vi "Double FFT Mesurament (Max Bin detection - Control - Init Wave&Window - Snapshot - DoubleFFT) RT Test.vi"() -> ()   [LabVIEW 2014]
uses:
  <vilib>/Platform/TimedLoop/XDataNode/timing_clust.ctl
  <vilib>/Platform/TimedLoop/XDataNode/nitl_modes.ctl
  <vilib>/Platform/TimedLoop/XDataNode/wakeup.ctl
  <vilib>/FPGAPlugInAG/sbRIO-9636/niLvFpga_Open_sbRIO-9636.vi
  <vilib>/rvi/interface/common/dynamic/niFpgaDynamicAddResources.vi
  <vilib>/Utility/error.llb/Error Cluster From Error Code.vi
  <vilib>/rvi/errors/niLvFpgaAdjustHostInterfaceError.vi
  <vilib>/rvi/interface/common/niFpgaWaitOnOcc.vi
  <vilib>/FPGAPlugInAG/Dynamic/niLvFpga_Run_Dynamic.vi
  <vilib>/FPGAPlugInAG/Dynamic/niLvFpga_Abort_Dynamic.vi
  <vilib>/FPGAPlugInAG/Dynamic/niLvFpga_Reset_Dynamic.vi
  <vilib>/FPGAPlugInAG/Dynamic/niLvFpga_Close_Dynamic.vi
  <vilib>/rvi/interface/nirviOpenFPGA/nirviOpenFPGA.xnode
  FPGA Bitfiles/LaserDistanceSen_FPGATarget_DoubleFFTMesuram_TCh4DSruzm8.lvbitx
  FPGA Target/Test VIs/Double FFT Mesurament (Max Bin detection - Control - Init Wave&Window - Snapshot - DoubleFFT) test.vi
  <vilib>/rvi/interface/nirviReadWriteControl/nirviReadWriteControl.xnode
  <vilib>/rvi/interface/nirviMethod/nirviMethod.xnode
  <vilib>/Platform/TimedLoop/XDataNode/XDataNode.xnode
  <vilib>/rvi/interface/nirviCloseFPGA/nirviCloseFPGA.xnode
  <vilib>/FPGAPlugInAG/Dynamic/niLvFpga_ConfigureFifo_Dynamic.vi
  <vilib>/rvi/errors/niLvFpgaMergeErrorWithErrorCode.vi
  <vilib>/FPGAPlugInAG/Dynamic/niLvFpga_StartFifo_Dynamic.vi
  <vilib>/rvi/interface/Simulation/niFpgaSimulationCallBeginRW.vi
  <vilib>/FPGAPlugInAG/Dynamic/niLvFpga_ReadFifo_Dynamic.vi
  <vilib>/Platform/TimedLoop/XDataNode/XDNodeRunTimeDep.lvlib
  NiFpgaLv.dll
panel:
  out "Second FFT (bin)":dbl[](graph)
  out "Second Signal (points) - Rising Triangular":dbl[](graph)
  out "Elements Remaining FFT":u32
  out "Elements Remaining Signal":u32
  out "First FFT (bin)":dbl[](graph)
  out "First Signal (points) - Falling Triangular":dbl[](graph)
  in  "Snapshot":bool
  in  "Windowing":T1(ring)
  in  "first bin":i32=10
  in  "last bin":i32=255
  in  "lower limit 2":u32(slide)=677 scale=625.0..738.0
  in  "lower limit 1":u32(slide)=59 scale=0.0..113.0
  out "Detected Frequency Tone - (Hz)":dbl
  in  "stop":bool
  out "Max Bin":i32
  out "Max Amp":dbl format="%.2f"
  out "Prev Bin":i32
  out "Next Bin":i32
  out "Prev Amp":dbl format="%.2f"
  out "Next Amp":dbl format="%.2f"
  out "Interpolated Bin":dbl
  in  "Interpolation Method":T2(ring)=enum."Jain"
  # "WARNING:\nOnce pressed wait untill the end of operation"
  # "ONLINE parameter"
  # "OFFLINE parameters"
  # "Max Detection FFT bin range"
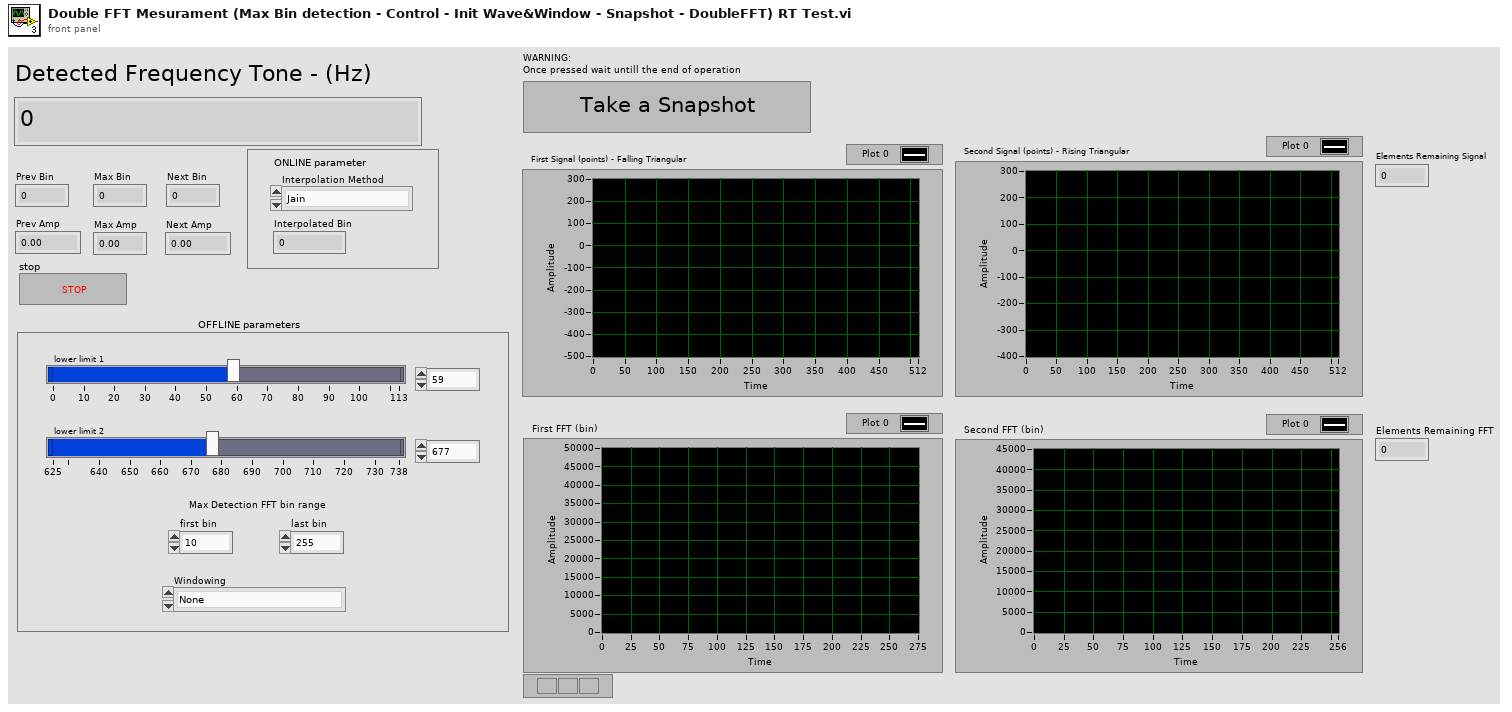
[diagram p1: front panel]
types:
  T1 = enum16{"None", "Hanning", "Hamming", "Blackman", "Blackman-Harris"}
  T2 = enum16{"Quadratic", "McLeodd", "Barycentric", "Jain"}
  T3 = typedef "XDNodeRunTimeDep.lvlib/timing_clust.ctl" = cluster{"Expected End [f-1]":u64, "Actual End [f-1]":u64, "Finished Late? [f-1]":bool, "Expected End [i-1]":u64, "Actual End [i-1]":u64, "Finished Late? [i-1]":bool, "Expected Start [i]":u64, "Actual Start [i]":u64, "Expected Start [f]":u64, "Actual Start [f]":u64, "Source Name":string, "Structure Name":string, "Period":i64, "Deadline":i64, "Offset":i64, "Start":i64, "Priority":i32, "Timeout":i32, "Mode":T4, "Wakeup Reason":T5, "Error":errorcluster, "Source Type":string, "Secondary Source Type":string, "Global End Time":u64, "Global Start Time":u64, "Frame Duration":u64, "Iteration Duration":u64, "Assigned CPU":i32, "I/O Scan Engine Mode":u32}
  T4 = typedef "XDNodeRunTimeDep.lvlib/nitl_modes.ctl" = enum32{"No Change", "Process missed periods, maintain original phase", "Discard missed periods, maintain original phase", "Process missed periods, ignore original phase", "Discard missed periods, ignore original phase"}
  T5 = typedef "XDNodeRunTimeDep.lvlib/wakeup.ctl" = enum32{"Normal", "Aborted", "Asynchronous wakeup", "Timing source error", "Timed loop error", "Timeout"}
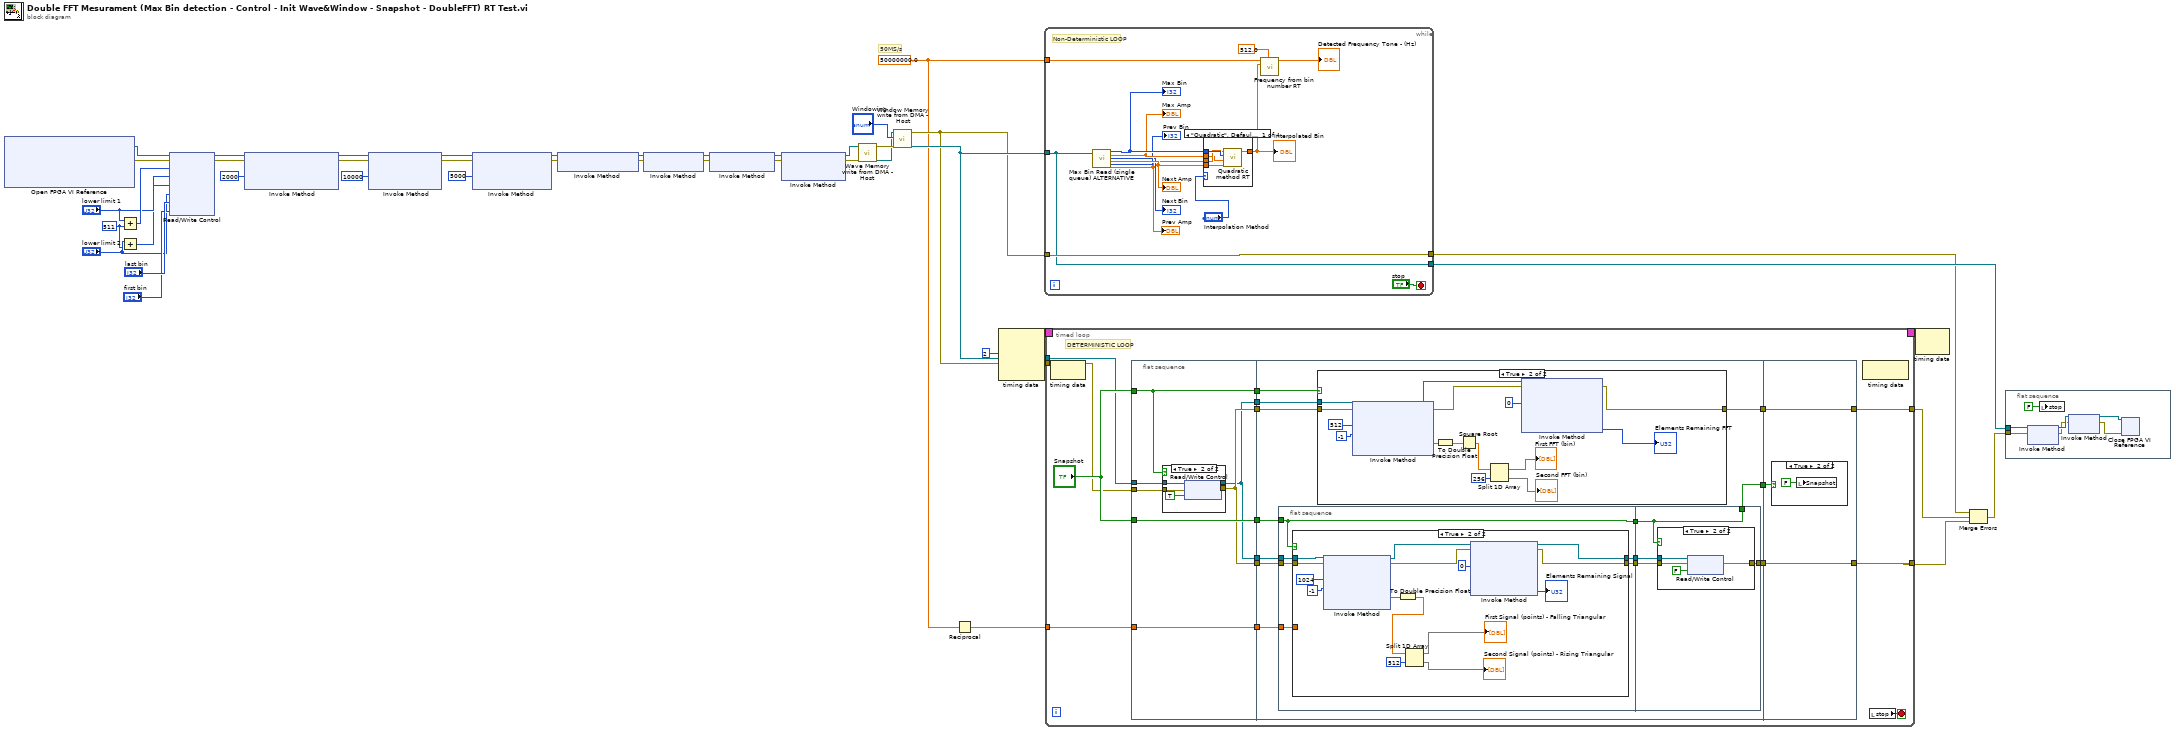
[diagram p0: block diagram]
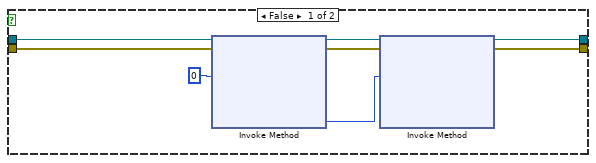
[diagram p3: hidden frame]
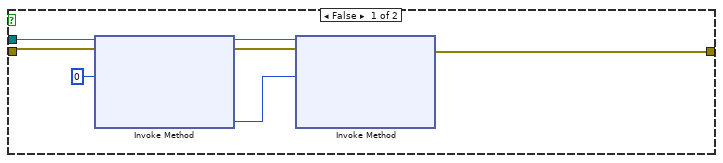
[diagram p5: hidden frame]
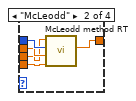
[diagram p7: hidden frame]
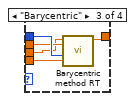
[diagram p8: hidden frame]
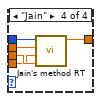
[diagram p9: hidden frame]
diagram:
  w37 = u32 511 ("y")
  w15 = 50000000.0 ("Sample Rate (S/s)")
  # "50MS/s"
  n1 = xnode "Open FPGA VI Reference"() -> ("FPGA VI Reference Out"=w36:refnum<k20>, "error out"=w35:errorcluster)  [unwired: 2 in]
  n2 = Add(x="lower limit 1", y=w37) -> (x+y=w41:u32)
  n3 = Add(x="lower limit 2", y=w37) -> (x+y=w39:u32)
  n4 = xnode "Read/Write Control"("FPGA VI Reference In"=w36, "error in"=w35, "upper limit 1"=w41, "upper limit 2"=w39, "lower limit 1"="lower limit 1", "lower limit 2"="lower limit 2", "last bin"="last bin", "first bin"="first bin") -> ("FPGA VI Reference Out"=w30:refnum<k20>, "error out"=w29:errorcluster)
  n5 = xnode "Invoke Method"("FPGA VI Reference In"=w30, "error in"=w29, "Requested Depth"=u32 2000) -> ("FPGA VI Reference Out"=w28:refnum<k20>, "error out"=w27:errorcluster)  [unwired: 1 out]
  n6 = xnode "Invoke Method"("FPGA VI Reference In"=w28, "error in"=w27, "Requested Depth"=u32 10000) -> ("FPGA VI Reference Out"=w26:refnum<k20>, "error out"=w25:errorcluster)  [unwired: 1 out]
  n7 = xnode "Invoke Method"("FPGA VI Reference In"=w26, "error in"=w25, "Requested Depth"=u32 5000) -> ("FPGA VI Reference Out"=w9:refnum<k20>, "error out"=w10:errorcluster)  [unwired: 1 out]
  n8 = xnode "Invoke Method"("FPGA VI Reference In"=w9, "error in"=w10) -> ("FPGA VI Reference Out"=w19:refnum<k20>, "error out"=w18:errorcluster)
  n9 = xnode "Invoke Method"("FPGA VI Reference In"=w19, "error in"=w18) -> ("FPGA VI Reference Out"=w21:refnum<k20>, "error out"=w20:errorcluster)
  n10 = xnode "Invoke Method"("FPGA VI Reference In"=w21, "error in"=w20) -> ("FPGA VI Reference Out"=w7:refnum<k20>, "error out"=w8:errorcluster)
  n11 = xnode "Invoke Method"("FPGA VI Reference In"=w7, "error in"=w8) -> ("FPGA VI Reference Out"=w14:refnum<k20>, "error out"=w13:errorcluster)  [unwired: 1 in]
  n12 = call "Wave Memory write from DMA - Host.vi"("error in"=w13, "FPGA VI Reference In"=w14) -> ("FPGA VI Reference Out"=w11:refnum<k20>, "error out"=w12:errorcluster)  [unwired: 7 in, 1 out]
  n13 = call "Window Memory write from DMA - Host.vi"("error in"=w12, "Enum"="Windowing", "FPGA VI Reference In"=w11) -> ("FPGA VI Reference Out"=w32:refnum<k20>, "error out"=w31:errorcluster)  [unwired: 5 in, 2 out]
  n14 = Reciprocal(x=w15) -> (1/x=w16:dbl)
  n15 = node-c288(i64 2 ("Period")) -> (w6:T3)  [unwired: 3 in]
  n16 = while {
    tunnel: w15 -> [w56]
    tunnel: w32 -> [w54]
    tunnel: w31 -> [w55]
    tunnel: [w54] -> w34
    tunnel: [w55] -> w2
    stop <- "stop" stop-if-true
    # "Non-Deterministic LOOP"
    n17 = call "Max Bin Read (single queue) ALTERNATIVE.vi"("FPGA VI Reference In"=w54) -> ("Max Bin"=w50:i32, "Max Amp"=w49:dbl, "Next Bin"=→"Next Bin":i32, "Next Amp"=w48:dbl, "Prev Bin"=→"Prev Bin":i32, "Prev Amp"=w47:dbl)  [unwired: 12 in, 1 out]
    "Max Bin" <- w50
    "Max Amp" <- w49
    "Prev Amp" <- w47
    "Next Amp" <- w48
    n18 = case shown="\"Quadratic\", Default" "Interpolation Method" {
      tunnel: w50 -> [w61 w66 w71 w76]
      tunnel: w49 -> [w58 w65 w70 w75]
      tunnel: w47 -> [w59 w64 w69 w74]
      tunnel: w48 -> [w60 w63 w68 w73]
      tunnel: [w62 w67 w72 w77] -> w51
      frame "Quadratic", Default {
        n19 = call "Quadratic method RT.vi"("Next Amplitude"=w60, "Max Amplitude"=w58, "Max bin"=w61, "Prev Amplitude"=w59) -> ("Bin"=w62:dbl)  [unwired: 7 in]
      }
      frame "McLeodd" {
        n20 = call "McLeodd method RT.vi"("Next Amp"=w63, "Max Amp"=w65, "Max Bin"=w66, "Prev Amp"=w64) -> ("Bin"=w67:dbl)  [unwired: 7 in]
      }
      frame "Barycentric" {
        n21 = call "Barycentric method RT.vi"("Next Amp"=w68, "Max Bin"=w71, "Max Amp"=w70, "Prev Amp"=w69) -> ("Bin"=w72:dbl)  [unwired: 7 in]
      }
      frame "Jain" {
        n22 = call "Jain's method RT.vi"("Prev Amp"=w74, "Next Amp"=w73, "Max Amp"=w75, "Max Bin"=w76) -> ("Bin"=w77:dbl)  [unwired: 7 in]
      }
    }
    "Interpolated Bin" <- w51
    n23 = call "Frequency from bin number RT.vi"("FFT size"=512.0, "Bin number"=w51, "Sample Rate (S/s)"=w56) -> ("Detected Frequency (Hz)"=→"Detected Frequency Tone - (Hz)":dbl)  [unwired: 8 in]
  }
  n24 = timed-loop {
    tunnel: w32 -> [w88]
    tunnel: w31 -> [w89]
    tunnel: [w91] -> w3
    tunnel: w16 -> [w93]
    tunnel: [w92] -> w1
    timing: w6 -> [_]
    timing-out: [_] -> w5
    stop <- w94 stop-if-true
    # "DETERMINISTIC LOOP"
    n25 = node-c288() -> ()  [unwired: 1 in, 1 out]
    n26 = flat-sequence {
      tunnel: w88 -> [w99]
      tunnel: w89 -> [w100]
      tunnel: "Snapshot" -> [w97]
      tunnel: "Snapshot" -> [w102]
      tunnel: w93 -> [w103]
      tunnel: [w101] -> w87
      tunnel: [w103] -> w86
      tunnel: [w102] -> w85
      tunnel: [w97] -> w84
      tunnel: [w101] -> w83
      tunnel: [w98] -> w82
      tunnel: [w98] -> w81
      tunnel: w87 -> [w119]
      tunnel: w86 -> [w118]
      tunnel: w85 -> [w112]
      tunnel: w84 -> [w115]
      tunnel: w83 -> [w114]
      tunnel: w82 -> [w113]
      tunnel: w81 -> [w120]
      tunnel: [w117] -> w80
      tunnel: [w116] -> w79
      tunnel: [w111] -> w78
      tunnel: [w185] -> w91
      tunnel: [w186] -> w92
      tunnel: w80 -> [w186]
      tunnel: w79 -> [w185]
      tunnel: w78 -> [w184]
      frame #0 {
        n27 = case shown="True" w97 {
          tunnel: [w104 w109] -> w101
          tunnel: w100 -> [w104 w108]
          tunnel: w99 -> [w105 w107]
          tunnel: [w105 w106] -> w98
          frame False {
          }
          frame True {
            n28 = xnode "Read/Write Control"("FPGA VI Reference In"=w107, "error in"=w108, "snapshot"=TRUE) -> ("FPGA VI Reference Out"=w106:refnum<k20>, "error out"=w109:errorcluster)
          }
        }
      }
      frame #1 {
        n29 = flat-sequence {
          tunnel: w120 -> [w129]
          tunnel: w119 -> [w128]
          tunnel: w118 -> [w127]
          tunnel: w112 -> [w124]
          tunnel: [w126] -> w123
          tunnel: [w125] -> w122
          tunnel: [w124] -> w121
          tunnel: [w154] -> w116
          tunnel: w123 -> [w156]
          tunnel: w122 -> [w155]
          tunnel: w121 -> [w153]
          tunnel: [w153] -> w111
          frame #0 {
            n30 = case shown="True" w124 {
              tunnel: w129 -> [w136 w152]
              tunnel: w128 -> [w134 w151]
              tunnel: [w133 w144] -> w125
              tunnel: w127 -> [_ _]
              tunnel: [w130 w143] -> w126
              frame False {
                n31 = xnode "Invoke Method"("FPGA VI Reference In"=w136, "error in"=w134, "Number of Elements"=u32 0) -> ("FPGA VI Reference Out"=w132:refnum<k20>, "error out"=w131:errorcluster, "Elements Remaining"=w135:u32)  [unwired: 1 in, 1 out]
                n32 = xnode "Invoke Method"("FPGA VI Reference In"=w132, "error in"=w131, "Number of Elements"=w135) -> ("FPGA VI Reference Out"=w130:refnum<k20>, "error out"=w133:errorcluster)  [unwired: 1 in, 2 out]
              }
              frame True {
                n33 = xnode "Invoke Method"("FPGA VI Reference In"=w152, "error in"=w151, "Number of Elements"=u32 1024, "Timeout (ms)"=-1) -> ("FPGA VI Reference Out"=w146:refnum<k20>, "error out"=w145:errorcluster, "Data"=w148:fxp<+/-,12,12>[])  [unwired: 1 out]
                n34 = To Double Precision Float(number=w148) -> (double precision float=w141:dbl[])
                n35 = Split 1D Array(array=w141, index=512) -> (first subarray=→"First Signal (points) - Falling Triangular":dbl[], second subarray=→"Second Signal (points) - Rising Triangular":dbl[])
                n36 = xnode "Invoke Method"("FPGA VI Reference In"=w146, "error in"=w145, "Number of Elements"=u32 0) -> ("FPGA VI Reference Out"=w143:refnum<k20>, "error out"=w144:errorcluster, "Elements Remaining"=→"Elements Remaining Signal":u32)  [unwired: 1 in, 1 out]
              }
            }
          }
          frame #1 {
            n37 = case shown="True" w153 {
              tunnel: [w157 w159] -> w154
              tunnel: w156 -> [_ w160]
              tunnel: w155 -> [w157 w158]
              frame False {
              }
              frame True {
                n38 = xnode "Read/Write Control"("FPGA VI Reference In"=w160, "error in"=w158, "snapshot"=FALSE) -> ("error out"=w159:errorcluster)  [unwired: 1 out]
              }
            }
          }
        }
        n39 = case shown="True" w115 {
          tunnel: w113 -> [w167 w178]
          tunnel: w114 -> [w164 w179]
          tunnel: [w163 w177] -> w117
          frame False {
            n40 = xnode "Invoke Method"("FPGA VI Reference In"=w167, "error in"=w164, "Number of Elements"=u32 0) -> ("FPGA VI Reference Out"=w165:refnum<k20>, "error out"=w162:errorcluster, "Elements Remaining"=w166:u32)  [unwired: 1 in, 1 out]
            n41 = xnode "Invoke Method"("FPGA VI Reference In"=w165, "error in"=w162, "Number of Elements"=w166) -> ("error out"=w163:errorcluster)  [unwired: 1 in, 3 out]
          }
          frame True {
            n42 = xnode "Invoke Method"("FPGA VI Reference In"=w178, "error in"=w179, "Number of Elements"=u32 512, "Timeout (ms)"=-1) -> ("FPGA VI Reference Out"=w175:refnum<k20>, "error out"=w176:errorcluster, "Data"=w181:fxp<+,44,44>[])  [unwired: 1 out]
            n43 = To Double Precision Float(number=w181) -> (double precision float=w180:dbl[])
            n44 = Square Root(x=w180) -> (sqrt(x)=w170:dbl[])
            n45 = Split 1D Array(array=w170, index=256) -> (first subarray=→"First FFT (bin)":dbl[], second subarray=→"Second FFT (bin)":dbl[])
            n46 = xnode "Invoke Method"("FPGA VI Reference In"=w175, "error in"=w176, "Number of Elements"=u32 0) -> ("error out"=w177:errorcluster, "Elements Remaining"=→"Elements Remaining FFT":u32)  [unwired: 1 in, 2 out]
          }
        }
      }
      frame #2 {
        n47 = case shown="True" w184 {
          frame False {
          }
          frame True {
            n48 = local write "Snapshot"(FALSE ("Snapshot")) -> ()
          }
        }
      }
    }
    n49 = node-c288() -> ()  [unwired: 1 in, 1 out]
    n50 = local read "stop"() -> (w94:bool)
  }
  n51 = node-c288(w5) -> ()  [unwired: 1 out]
  n52 = Merge Errors(w2, w1, w3) -> (w17:errorcluster)
  n53 = flat-sequence {
    tunnel: w34 -> [w194]
    tunnel: w17 -> [w193]
    frame #0 {
      n54 = xnode "Invoke Method"("FPGA VI Reference In"=w194, "error in"=w193) -> ("FPGA VI Reference Out"=w189:refnum<k20>, "error out"=w188:errorcluster)
      n55 = local write "stop"(FALSE ("stop")) -> ()
      n56 = xnode "Invoke Method"("FPGA VI Reference In"=w189, "error in"=w188) -> ("FPGA VI Reference Out"=w190:refnum<k20>, "error out"=w191:errorcluster)
      n57 = xnode "Close FPGA VI Reference"("FPGA VI Reference In"=w190, "error in"=w191) -> ()  [unwired: 1 out]
    }
  }
